vi "Check_Module_Information.vi"(0 "Address Cluster":T1 {"tsl_communcation_method" items=["GPIB", "C232C", "TCPIP", "USB"]; "MPM_communcation_method" items=["GPIB", "C232C", "TCPIP", "USB"]}, 3 "错误输入（无错误）":errorcluster caption="error in") -> (7 "Address Cluster out":T1 {"tsl_communcation_method" items=["GPIB", "C232C", "TCPIP", "USB"]; "MPM_communcation_method" items=["GPIB", "C232C", "TCPIP", "USB"]}, 8 "Flag_215":bool, 9 "Flag_213":bool, 10 "error out":errorcluster)   [LabVIEW 2017]
doc: "check Module information inside system"
uses:
  CTL/Address Cluster.ctl
  D:/test/ILSTS/LV_IL/LV_IL_Sample_x86/DLL/InstrumentDLL.dll
  DLL/InstrumentDLL.dll
  Share/PowerMonitorType.vi
panel:
  in  "counter_215":i32
  in  "enable_module_count":i32
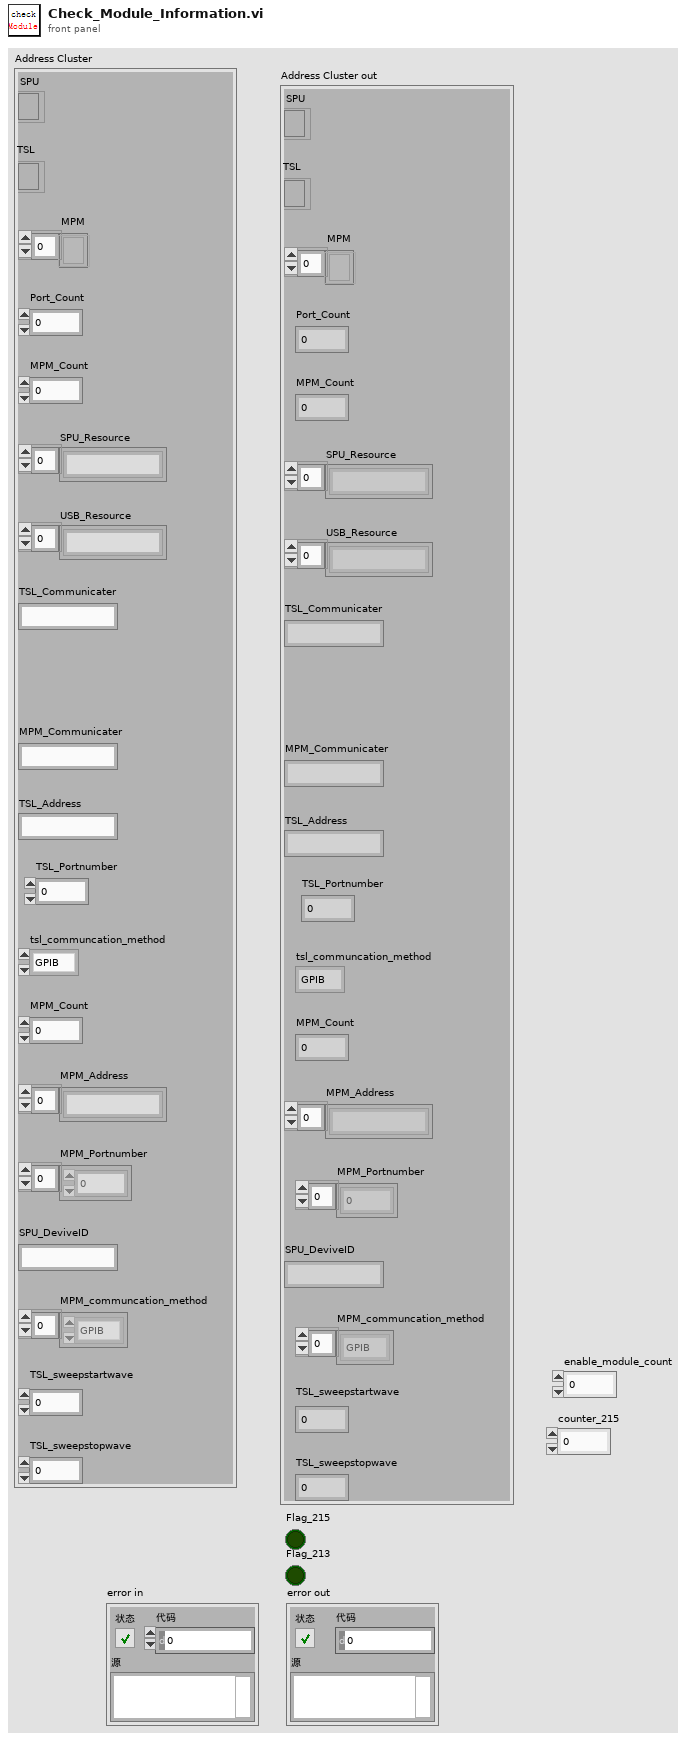
[diagram p1: front panel]
types:
  T1 = typedef "Address Cluster.ctl" = cluster{"SPU":refnum<k24>, "MPM":refnum<k24>[], "Port_Count":dbl, "MPM_Count":dbl, "SPU_Resource":string[], "USB_Resource":string[], "MPM_Communicater":string, "MPM_Count":dbl, "MPM_Address":string[], "MPM_Portnumber":dbl[], "SPU_DeviveID":string, "MPM_communcation_method":i32[], "TSL_sweepstartwave":dbl, "TSL_sweepstopwave":dbl, "TSL_Address":string, "TSL_Communicater":string, "TSL":refnum<k24>, "tsl_communcation_method":i32, "TSL_Portnumber":dbl}
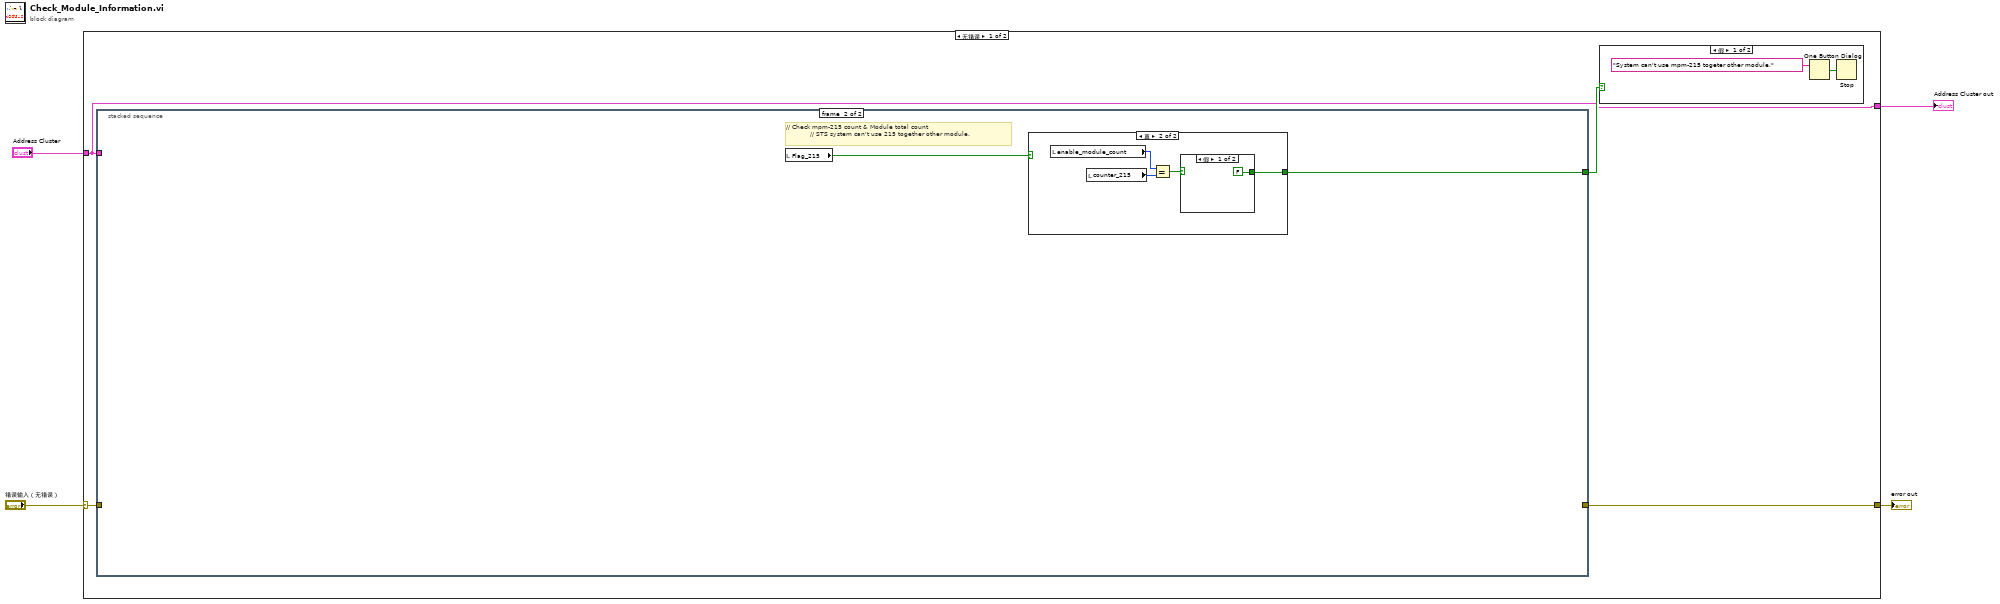
[diagram p0: block diagram]
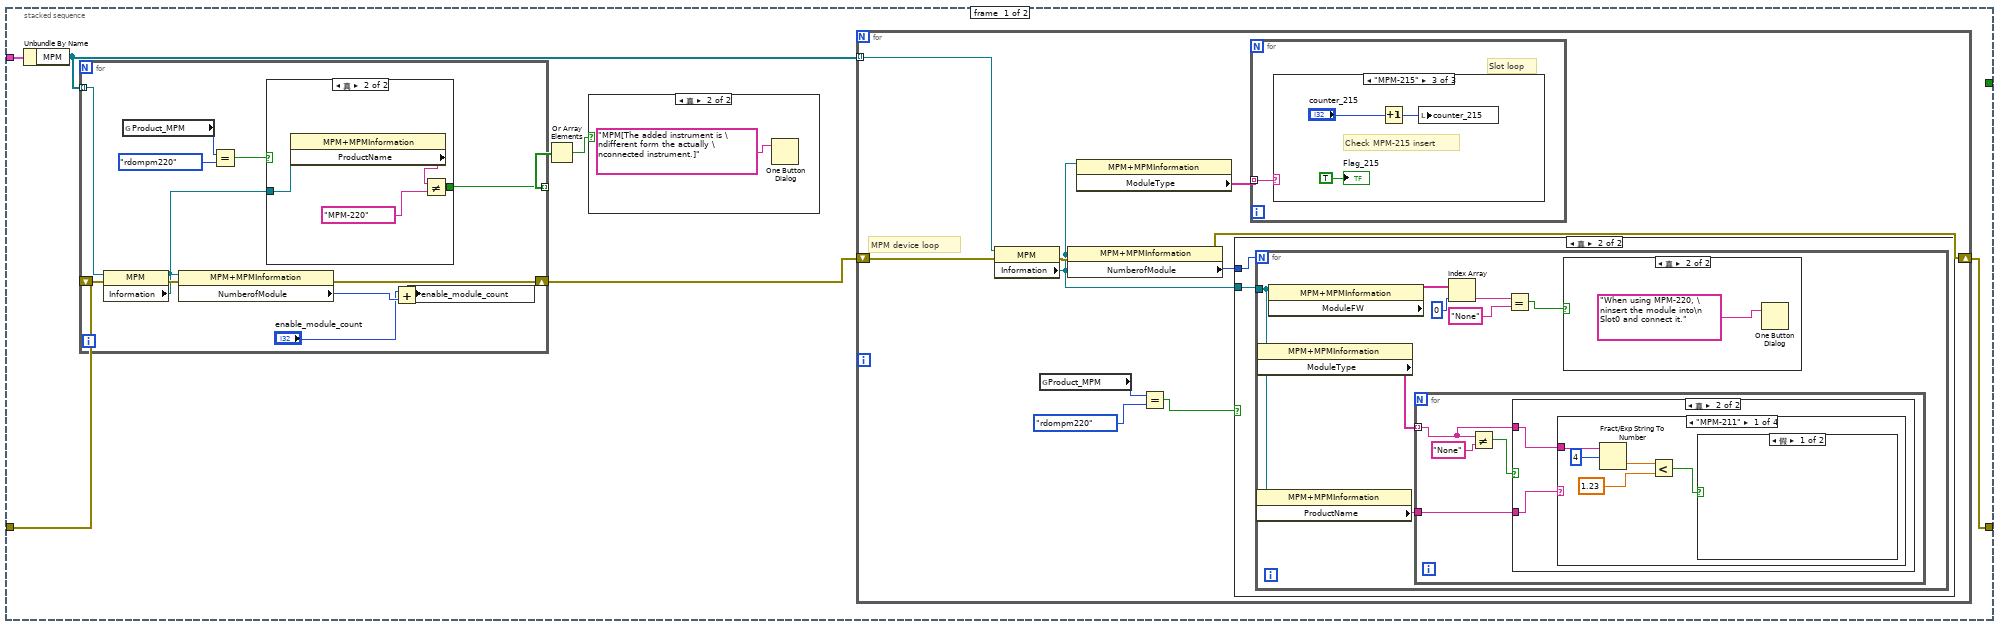
[diagram p3: hidden frame]
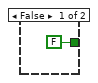
[diagram p5: hidden frame]
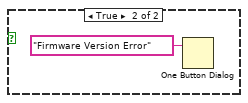
[diagram p8: hidden frame]
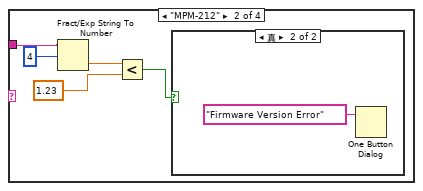
[diagram p9: hidden frame]
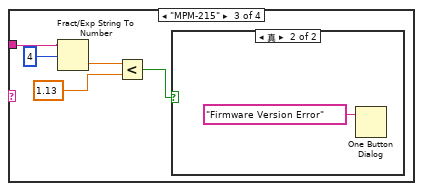
[diagram p11: hidden frame]
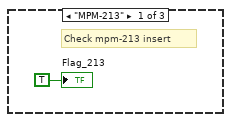
[diagram p15: hidden frame]
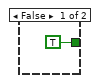
[diagram p17: hidden frame]
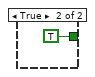
[diagram p18: hidden frame]
diagram:
  n1 = case shown="无错误" "错误输入（无错误）" {
    selector: "错误输入（无错误）" -> [w7 w96]
    tunnel: "Address Cluster" -> [w5 w95]
    tunnel: [w6 w96] -> w2
    tunnel: [w5 w95] -> w1
    frame No Error {
      n2 = stacked-sequence {
        tunnel: w5 -> [w17 _]
        tunnel: [_ w86] -> w8
        tunnel: w7 -> [w15 _]
        tunnel: [w13 _] -> w6
        frame #0 {
          n3 = Unbundle By Name(w17) -> ("MPM"=w16:refnum<k24>[])
          n4 = for {
            tunnel: w16 -> [w24] mode=indexing
            shift-right: [w25] -> w14
            shift-left: w15 -> [w27]
            tunnel: [w19] -> w12 mode=indexing
            n5 = property on="属性节点" class="MPM"(reference=w24, error in=w27) -> (error out=w26:errorcluster, "Information"=w20:refnum<k24>)  [unwired: 1 out]
            n6 = global read "PowerMonitorType.vi" "Product_MPM"() -> (w22:enum32{"rdompm210", "rdompm220"})
            n7 = property class="MPM+MPMInformation"(reference=w20, error in=w26) -> (error out=w25:errorcluster, "NumberofModule"=w30:i32)  [unwired: 1 out]
            n8 = Equal?(x=w22, y=enum32{"rdompm210", "rdompm220"}."rdompm220") -> (x = y?=w23:bool)
            n9 = case shown="真" w23 {
              tunnel: w20 -> [_ w35]
              tunnel: [FALSE w32] -> w19
              frame False {
              }
              frame True {
                n10 = property class="MPM+MPMInformation"(reference=w35) -> ("ProductName"=w34:string)  [unwired: 1 in, 2 out]
                n11 = Not Equal?(x=w34, y="MPM-220") -> (x != y?=w32:bool)
              }
            }
            n12 = Add(x="enable_module_count", y=w30) -> (x+y=w28:i32)
            n13 = local write "enable_module_count"(w28) -> ()
          }
          n14 = Or Array Elements(Boolean array=w12) -> (logical OR=w11:bool)
          n15 = case shown="真" w11 {
            frame False {
            }
            frame True {
              n16 = One Button Dialog(message="MPM[The added instrument is \ndifferent form the actually \nconnected instrument.]") -> ()  [unwired: 1 in, 1 out]
            }
          }
          n17 = for {
            tunnel: w16 -> [w45] mode=indexing
            shift-right: [w40] -> w13
            shift-left: w14 -> [w43]
            # "MPM device loop"
            n18 = property on="属性节点" class="MPM"(reference=w45, error in=w43) -> (error out=w41:errorcluster, "Information"=w39:refnum<k24>)  [unwired: 1 out]
            n19 = global read "PowerMonitorType.vi" "Product_MPM"() -> (w38:enum32{"rdompm210", "rdompm220"})
            n20 = property class="MPM+MPMInformation"(reference=w39, error in=w41) -> (error out=w40:errorcluster, "NumberofModule"=w42:i32)  [unwired: 1 out]
            n21 = property class="MPM+MPMInformation"(reference=w39) -> ("ModuleType"=w44:string[])  [unwired: 1 in, 2 out]
            n22 = Equal?(x=w38, y=enum32{"rdompm210", "rdompm220"}."rdompm220") -> (x = y?=w37:bool)
            n23 = case shown="真" w37 {
              tunnel: w42 -> [_ w47]
              tunnel: w39 -> [_ w46]
              frame False {
              }
              frame True {
                n24 = for {
                  N: w47 -> [_]
                  tunnel: w46 -> [w49]
                  n25 = property class="MPM+MPMInformation"(reference=w49) -> ("ProductName"=w48:string)  [unwired: 1 in, 2 out]
                  n26 = property class="MPM+MPMInformation"(reference=w49) -> ("ModuleType"=w50:string[])  [unwired: 1 in, 2 out]
                  n27 = property class="MPM+MPMInformation"(reference=w49) -> ("ModuleFW"=w55:string[])  [unwired: 1 in, 2 out]
                  n28 = for {
                    tunnel: w50 -> [w57] mode=indexing
                    tunnel: w48 -> [w56]
                    n29 = Not Equal?(x=w57, y="None") -> (x != y?=w58:bool)
                    n30 = case shown="真" w58 {
                      tunnel: w57 -> [_ w60]
                      tunnel: w56 -> [_ w61]
                      frame False {
                      }
                      frame True {
                        n31 = case shown="\"MPM-211\"" w61 {
                          tunnel: w60 -> [w66 w72 w78 _]
                          frame "MPM-211" {
                            n32 = Fract/Exp String To Number(string=w66, offset=4 ("offset (0)")) -> (number=w64:dbl)  [unwired: 2 in, 1 out]
                            n33 = Less?(x=w64, y=1.23) -> (x < y?=w62:bool)
                            n34 = case shown="假" w62 {
                              frame False {
                              }
                              frame True {
                                n35 = One Button Dialog(message="Firmware Version Error") -> ()  [unwired: 1 in, 1 out]
                              }
                            }
                          }
                          frame "MPM-212" {
                            n36 = Fract/Exp String To Number(string=w72, offset=4 ("offset (0)")) -> (number=w70:dbl)  [unwired: 2 in, 1 out]
                            n37 = Less?(x=w70, y=1.23) -> (x < y?=w68:bool)
                            n38 = case shown="真" w68 {
                              frame False {
                              }
                              frame True {
                                n39 = One Button Dialog(message="Firmware Version Error") -> ()  [unwired: 1 in, 1 out]
                              }
                            }
                          }
                          frame "MPM-215" {
                            n40 = Fract/Exp String To Number(string=w78, offset=4 ("offset (0)")) -> (number=w76:dbl)  [unwired: 2 in, 1 out]
                            n41 = Less?(x=w76, y=1.13) -> (x < y?=w74:bool)
                            n42 = case shown="真" w74 {
                              frame False {
                              }
                              frame True {
                                n43 = One Button Dialog(message="Firmware Version Error") -> ()  [unwired: 1 in, 1 out]
                              }
                            }
                          }
                          frame Default {
                          }
                        }
                      }
                    }
                  }
                  n44 = Index Array(array=w55, index=0) -> (element=w53:string)
                  n45 = Equal?(x=w53, y="None") -> (x = y?=w51:bool)
                  n46 = case shown="真" w51 {
                    frame False {
                    }
                    frame True {
                      n47 = One Button Dialog(message="When using MPM-220, \ninsert the module into\n Slot0 and connect it.") -> ()  [unwired: 1 in, 1 out]
                    }
                  }
                }
              }
            }
            n48 = for {
              tunnel: w44 -> [w81] mode=indexing
              # "Slot loop"
              n49 = case shown="\"MPM-215\"" w81 {
                frame "MPM-213" {
                  # "Check mpm-213 insert"
                  "Flag_213" <- TRUE ("Flag_213")
                }
                frame "MPM-211", Default {
                }
                frame "MPM-215" {
                  # "Check MPM-215 insert"
                  n50 = Increment(x="counter_215") -> (x+1=w83:i32)
                  n51 = local write "counter_215"(w83) -> ()
                  "Flag_215" <- TRUE ("Flag_215")
                }
              }
            }
          }
        }
        frame #1 {
          # "// Check mpm-215 count & Module total count\n            // STS system can't use 215 together other module."
          n52 = local read "Flag_215"() -> (w87:bool)
          n53 = case shown="真" w87 {
            tunnel: [TRUE w89] -> w86
            frame False {
            }
            frame True {
              n54 = local read "enable_module_count"() -> (w92:i32)
              n55 = local read "counter_215"() -> (w91:i32)
              n56 = Equal?(x=w92, y=w91) -> (x = y?=w90:bool)
              n57 = case shown="假" w90 {
                tunnel: [FALSE TRUE] -> w89
                frame False {
                }
                frame True {
                }
              }
            }
          }
        }
      }
      n58 = case shown="假" w8 {
        frame False {
          n59 = One Button Dialog(message="System can't use mpm-215 togeter other module." ("消息")) -> (true=w9:bool)  [unwired: 1 in]
          n60 = Stop(stop? (T)=w9) -> ()
        }
        frame True {
        }
      }
    }
    frame Error {
    }
  }
  "Address Cluster out" <- w1
  "error out" <- w2
